vi "Run greeter_client.vi"() -> ()   [LabVIEW 2019, in "helloworld_client.lvlib"]
uses:
  helloworld_client.lvlib
  RPC Messages/helloworld_HelloRequest.ctl
  RPC Messages/helloworld_HelloReply.ctl
panel:
  out "Response Data":T1
  in  "Request Data":T2={"name"="John"}
  out "error out":errorcluster
  in  "error in":errorcluster
  in  "Server Address":string="localhost:50051"
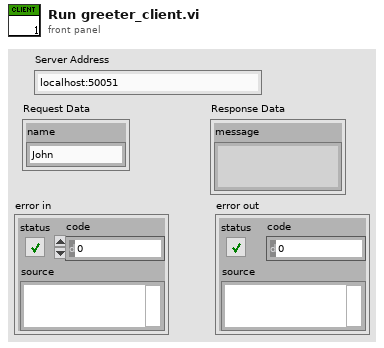
[diagram p1: front panel]
types:
  T1 = typedef "helloworld_client.lvlib/helloworld_HelloReply.ctl" = cluster{"message":string}
  T2 = typedef "helloworld_client.lvlib/helloworld_HelloRequest.ctl" = cluster{"name":string}
  T3 = typedef "grpc-lvsupport-release.lvlib/grpcId.ctl" = u64
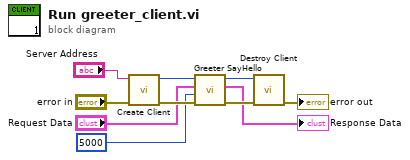
[diagram p0: block diagram]
diagram:
  n1 = call "Create Client.vi"("error in"="error in", "address"="Server Address") -> ("error out"=w7:errorcluster, "gRPC ID Out"=w8:T3)  [unwired: 8 in]
  n2 = call "Greeter SayHello.vi"("error in"=w7, "timeout (ms)"=5000, "Request Data"="Request Data", "gRPC ID"=w8) -> ("error out"=w5:errorcluster, "Response Data"=→"Response Data":T1, "gRPC ID out"=w6:T3)  [unwired: 5 in]
  n3 = call "Destroy Client.vi"("error in"=w5, "gRPC ID"=w6) -> ("error out"=→"error out":errorcluster)  [unwired: 9 in]
